vi "Initialize.vi"(8 "error in (no error)":errorcluster, 9 "top file info":string, 10 "swt file info":string) -> (0 "error out":errorcluster, 3 "Route Manager out":refnum<class "Route Manager.lvclass">)   [LabVIEW 2015, in "Route Manager.lvclass"]
uses:
  Route Manager.lvclass
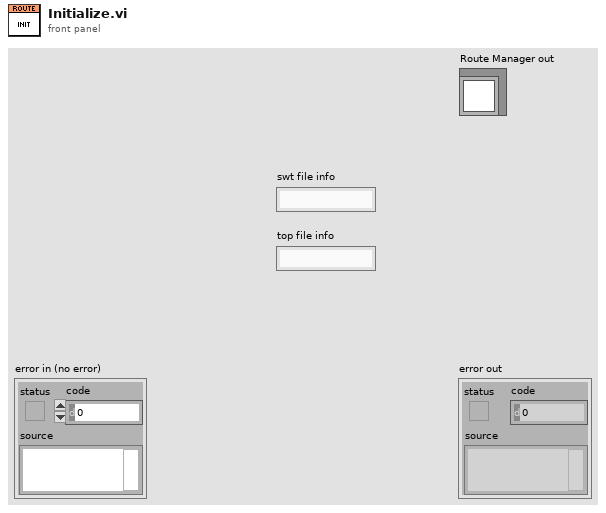
[diagram p1: front panel]
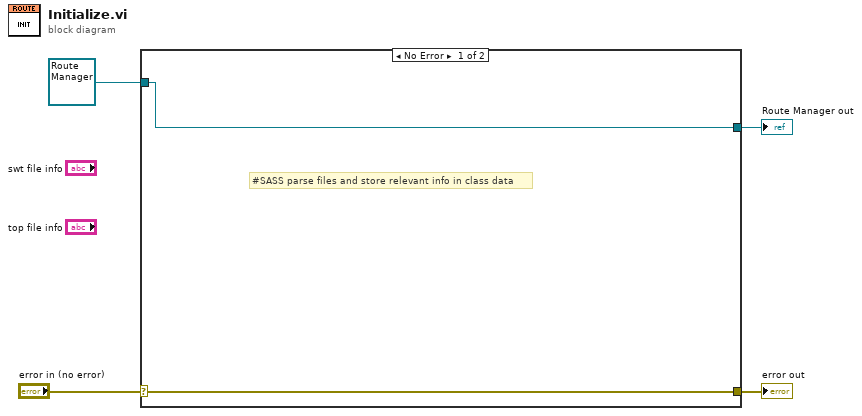
[diagram p0: block diagram]
diagram:
  n1 = case shown="No Error" "error in (no error)" {
    selector: "error in (no error)" -> [w6 w8]
    tunnel: [w6 w8] -> w3
    tunnel: refnum<class "Route Manager.lvclass"> refnum ("Route Manager out") -> [w5 w7]
    tunnel: [w5 w7] -> w1
    frame No Error {
      # "#SASS parse files and store relevant info in class data"
    }
    frame Error {
    }
  }
  "error out" <- w3
  "Route Manager out" <- w1
